vi "Example.vi"() -> ()   [LabVIEW 2016, in "斯坦道氨氮.lvlib"]
uses:
  Implementations/Listbox/Listbox.lvclass
  Implementations/Listbox Item/Listbox Item.lvclass
  Implementations/Listbox Item/Listbox Item.lvclass/Listbox Item.ctl
  Implementations/Listbox/Listbox.lvclass/Listbox.ctl
panel:
  in  "Stop Button":bool
  in  "Move to Left":bool
  in  "Move to Right":bool
  in  "Right Listbox":i32(listbox)
  in  "Left Listbox":i32(listbox)
  # "NOTICE -- YOU MUST LEAVE THIS NOTICE IN PLACE.\n\nCopyright (c) 2017, LIANG LIU Shawn.Liu.cn@gmail.com\nAll rights reserved.\n\nRedistribution and use in source and binary forms, with or without modification, are permitted provided that the following conditions are met:\n-Redistributions of source code must retain the above copyright notice, this list of conditions and the following disclaimer.\n-Redistributions in binary form must reproduce the above copyright notice, this list of conditions and the following disclaimer in the documentation and/or other materials provided with the distribution.\n-Neither the name of the eLp nor the names of its contributors may be used to endorse or promote products derived from this software without specific prior written permission.\n\nTHIS SOFTWARE IS PROVIDED BY THE COPYRIGHT HOLDERS AND CONTRIBUTORS \"AS IS\" AND ANY EXPRESS OR IMPLIED WARRANTIES, INCLUDING, BUT NOT LIMITED TO, THE IMPLIED WARRANTIES OF MERCHANTABILITY AND FITNESS FOR A PARTICULAR PURPOSE ARE DISCLAIMED. IN NO EVENT SHALL THE COPYRIGHT HOLDER OR CONTRIBUTORS BE LIABLE FOR ANY DIRECT, INDIRECT, INCIDENTAL, SPECIAL, EXEMPLARY, OR CONSEQUENTIAL DAMAGES (INCLUDING, BUT NOT LIMITED TO, PROCUREMENT OF SUBSTITUTE GOODS OR SERVICES; LOSS OF USE, DATA, OR PROFITS; OR BUSINESS INTERRUPTION) HOWEVER CAUSED AND ON ANY THEORY OF LIABILITY, WHETHER IN CONTRACT, STRICT LIABILITY, OR TORT (INCLUDING NEGLIGENCE OR OTHERWISE) ARISING IN ANY WAY OUT OF THE USE OF THIS SOFTWARE, EVEN IF ADVISED OF THE POSSIBILITY OF SUCH DAMAGE."
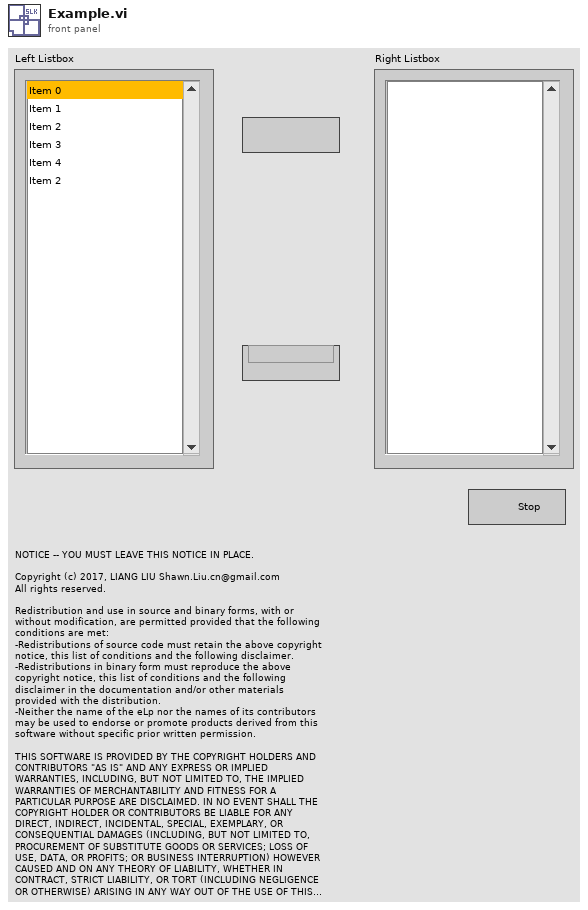
[diagram p1: front panel]
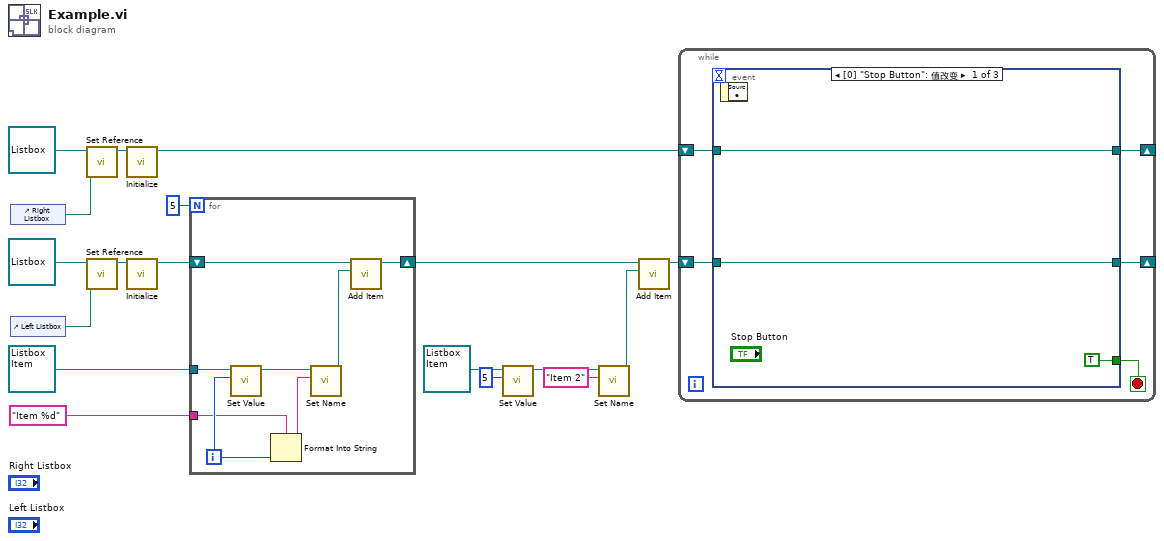
[diagram p0: block diagram]
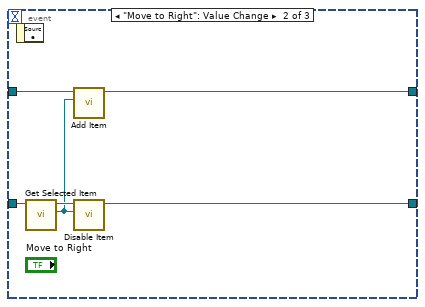
[diagram p2: hidden frame]
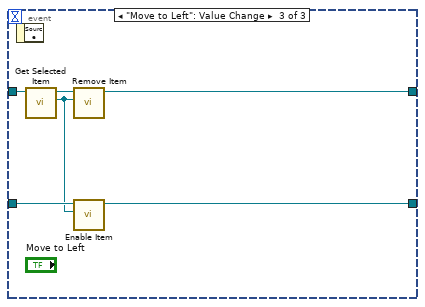
[diagram p3: hidden frame]
diagram:
  n1 = control-ref of="Right Listbox"() -> (w11:refnum<vi>)
  n2 = control-ref of="Left Listbox"() -> (w17:refnum<vi>)
  n3 = call "Set Reference.vi"("Reference"=w11, "Listbox in"=refnum<class "Listbox.lvclass"> refnum ("Listbox.lvclass")) -> ("Listbox out"=w9:refnum<class "Listbox.lvclass">)  [unwired: 9 in]
  n4 = call "Set Reference.vi"("Reference"=w17, "Listbox in"=refnum<class "Listbox.lvclass"> refnum ("Listbox.lvclass")) -> ("Listbox out"=w16:refnum<class "Listbox.lvclass">)  [unwired: 9 in]
  n5 = call-dynamic "Initialize.vi"("Listbox in"=w9) -> ("Listbox out"=w8:refnum<class "Listbox.lvclass">)  [unwired: 9 in, 1 out]
  n6 = call-dynamic "Initialize.vi"("Listbox in"=w16) -> ("Listbox out"=w10:refnum<class "Listbox.lvclass">)  [unwired: 9 in, 1 out]
  n7 = for {
    N: 5 -> [_]
    tunnel: refnum<class "Listbox Item.lvclass"> refnum ("Listbox Item.lvclass") -> [w25]
    shift-right: [w24] -> w7
    shift-left: w10 -> [w26]
    tunnel: "Item %d" ("format string") -> [w19]
    i -> [w21]
    n8 = call "Set Value.vi"("Value"=w21, "Listbox Item in"=w25) -> ("Listbox Item out"=w22:refnum<class "Listbox Item.lvclass">)  [unwired: 9 in]
    n9 = Format Into String(format string=w19, w21) -> (resulting string=w20:string)  [unwired: 2 in, 1 out]
    n10 = call "Set Name.vi"("Name"=w20, "Listbox Item in"=w22) -> ("Listbox Item out"=w23:refnum<class "Listbox Item.lvclass">)  [unwired: 9 in]
    n11 = call-dynamic "Add Item.vi"("Item"=w23, "Listbox in"=w26) -> ("Listbox out"=w24:refnum<class "Listbox.lvclass">)  [unwired: 8 in, 1 out]
  }
  n12 = call "Set Value.vi"("Value"=5, "Listbox Item in"=refnum<class "Listbox Item.lvclass"> refnum ("Listbox Item.lvclass")) -> ("Listbox Item out"=w5:refnum<class "Listbox Item.lvclass">)  [unwired: 9 in]
  n13 = call "Set Name.vi"("Name"="Item 2", "Listbox Item in"=w5) -> ("Listbox Item out"=w1:refnum<class "Listbox Item.lvclass">)  [unwired: 9 in]
  n14 = call-dynamic "Add Item.vi"("Item"=w1, "Listbox in"=w7) -> ("Listbox out"=w6:refnum<class "Listbox.lvclass">)  [unwired: 8 in, 1 out]
  n15 = while {
    shift-right: [w29] -> _
    shift-left: w8 -> [w31]
    shift-right: [w28] -> _
    shift-left: w6 -> [w30]
    stop <- w27 stop-if-true
    n16 = event shown="[0] \"Stop Button\": 值改变" {
      selector: _ -> [_ _ _]
      dyn-events: _ -> [_ _ _]
      timeout: _ -> [_ _ _]
      tunnel: w31 -> [w34 w39 w46]
      tunnel: w30 -> [w33 w40 w45]
      tunnel: [w34 w36 w43] -> w29
      tunnel: [w33 w37 w42] -> w28
      tunnel: [TRUE _ _] -> w27
      event "Stop Button": Value Change {
        n17 = event-data() -> ()  [unwired: 1 in, 1 out]
      }
      event "Move to Right": Value Change {
        n18 = event-data() -> ()  [unwired: 1 in, 1 out]
        n19 = call-dynamic "Get Selected Item.vi"("Listbox in"=w40) -> ("Item"=w35:refnum<class "Item.lvclass">, "Listbox out"=w38:refnum<class "Listbox.lvclass">)  [unwired: 8 in, 1 out]
        n20 = call-dynamic "Add Item.vi"("Item"=w35, "Listbox in"=w39) -> ("Listbox out"=w36:refnum<class "Listbox.lvclass">)  [unwired: 8 in, 1 out]
        n21 = call-dynamic "Disable Item.vi"("Item"=w35, "Listbox in"=w38) -> ("Listbox out"=w37:refnum<class "Listbox.lvclass">)  [unwired: 8 in, 1 out]
      }
      event "Move to Left": Value Change {
        n22 = event-data() -> ()  [unwired: 1 in, 1 out]
        n23 = call-dynamic "Get Selected Item.vi"("Listbox in"=w46) -> ("Item"=w41:refnum<class "Item.lvclass">, "Listbox out"=w44:refnum<class "Listbox.lvclass">)  [unwired: 8 in, 1 out]
        n24 = call-dynamic "Remove Item.vi"("Item"=w41, "Listbox in"=w44) -> ("Listbox out"=w43:refnum<class "Listbox.lvclass">)  [unwired: 8 in, 1 out]
        n25 = call-dynamic "Enable Item.vi"("Item"=w41, "Listbox in"=w45) -> ("Listbox out"=w42:refnum<class "Listbox.lvclass">)  [unwired: 8 in, 1 out]
      }
    }
  }
